vi "Logger.PGSQL.TestLauncher.vi"() -> ()   [LabVIEW 2019, in "Logger.PGSQL.lvclass"]
uses:
  Logger.PGSQL.lvclass
  <vilib>/JKI/JKI SMO/SMO/Typedefs/SMOState --Enum.ctl
  C:/Program Files (x86)/National Instruments/LabVIEW 2019/vi.lib/JKI/JKI SMO/SMO/SMO.lvclass
  C:/Users/patrick/Documents/GitHub/Instrument-Framework/lvsrc/SMOs/Logger/Logger.lvclass
  <vilib>/JKI/JKI SMO/SMO/SMO.lvclass/SMO.ctl
  <vilib>/JKI/JKI SMO/SMO/Private/ReftoDVR--SMO.vi
  <vilib>/JKI/JKI SMO/SMO/SMO.lvclass
  Logger/Logger.lvclass
panel:
  out "Data":variant
  out "x+1":i32=3
  out "time":u32
  out "read":u32
  out "write":u32=341910847
  in  "Address":string="llab_038:d005(TEST_TABLE--Columntest2())"
  in  "Write":bool
  in  "test value":dbl=2.0
  out "SMO State":T1=enum."Stopped"
  out "error out":errorcluster
  in  "Stop":bool
  # "Logger Test Launcher (postgreSQL)"
  # "For instructions on how to use the JKI State Machine Objects, examples and video tutorials, visit:\nhttp://jki.net/state-machine-objects/\n\nJKI State Machine Objects™\nhttp://jki.net/state-machine-objects/\nCopyright (C) 2005-2015, JKI <info@jki.net>\nALL RIGHTS RESERVED"
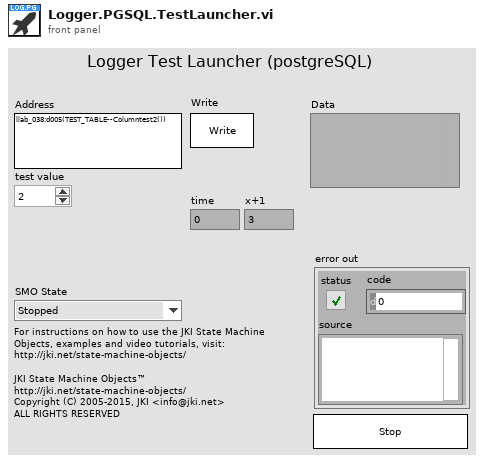
[diagram p1: front panel]
types:
  T1 = typedef "SMO.lvclass/SMOState --Enum.ctl" = enum16{"unknown", "Created", "Started", "Stopped"}
  T2 = typedef "SMO.lvclass/Public Events.ctl" = cluster{"Error":refnum<user-event>, "State":refnum<user-event>, "Reserve State":refnum<user-event>}
  T3 = typedef "Logger.PGSQL.lvclass/PublicEvents--Cluster.ctl" = cluster{"Read Variable":refnum<user-event>}
  T4 = cluster{"Event Registration Refnum":refnum<event-registration>}
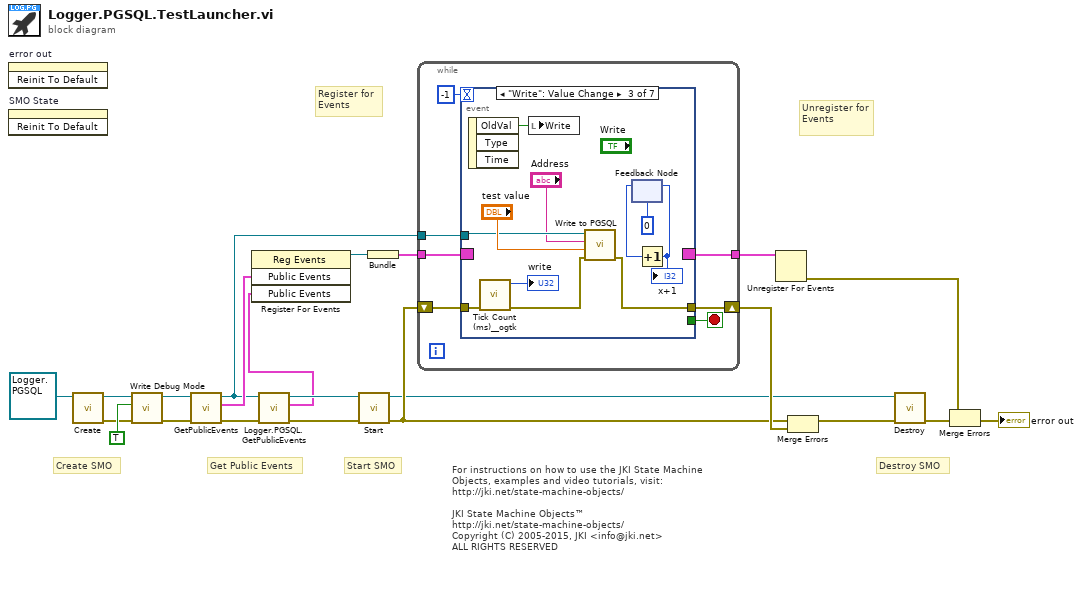
[diagram p0: block diagram]
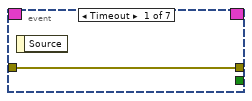
[diagram p2: hidden frame]
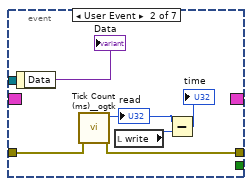
[diagram p3: hidden frame]
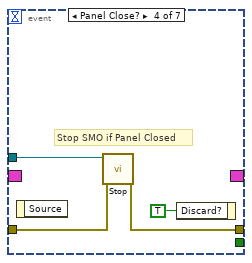
[diagram p4: hidden frame]
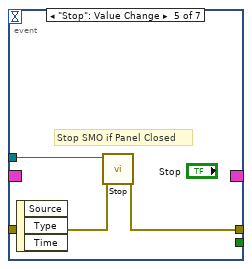
[diagram p5: hidden frame]
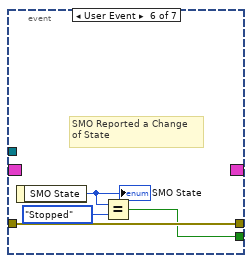
[diagram p6: hidden frame]
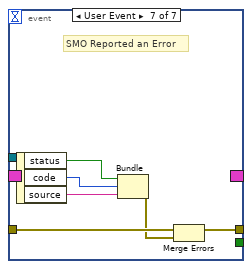
[diagram p7: hidden frame]
diagram:
  # "For instructions on how to use the JKI State Machine Objects, examples and video tutorials, visit:\nhttp://jki.net/state-machine-objects/\n\nJKI State Machine Objects™\nhttp://jki.net/state-machine-objects/\nCopyright (C) 2005-2015, JKI <info@jki.net>\nALL RIGHTS RESERVED"
  # "Get Public Events"
  # "Start SMO"
  # "Destroy SMO"
  # "Create SMO"
  # "Unregister for Events"
  # "Register for Events"
  n1 = invoke on="error out" class="Clust (strict)" method="Reinit To Default"() -> ()  [unwired: 3 in, 3 out]
  n2 = invoke on="SMO State" class="Enum (strict)" method="Reinit To Default"() -> ()  [unwired: 3 in, 3 out]
  n3 = call <vilib>:"Create.vi"("SMO"=refnum<class "Logger.PGSQL.lvclass"> refnum ("SMO.Template.lvclass")) -> ("error out"=w4:errorcluster, "SMO out"=w1:refnum<class "Logger.PGSQL.lvclass">)  [unwired: 8 in, 1 out]
  n4 = call "Write Debug Mode.vi"("error in (no error)"=w4, "Debug Mode?"=TRUE, "Logger in"=w1) -> ("error out"=w3:errorcluster, "Logger out"=w2:refnum<class "Logger.PGSQL.lvclass">)  [unwired: 7 in]
  n5 = call <vilib>:"GetPublicEvents.vi"("error in (no error)"=w3, "SMO"=w2) -> ("error out"=w9:errorcluster, "Public Events"=w12:T2, "SMO out"=w10:refnum<class "Logger.PGSQL.lvclass">)  [unwired: 7 in]
  n6 = call "Logger.PGSQL.GetPublicEvents.vi"("error in (no error)"=w9, "Logger"=w10) -> ("error out"=w8:errorcluster, "Public Events"=w6:T3, "Logger out"=w7:refnum<class "Logger.PGSQL.lvclass">)  [unwired: 7 in]
  n7 = register-events(w12, w6) -> (reference out=w11:refnum<event-registration>)  [unwired: 2 in, 1 out]
  n8 = call <vilib>:"Start.vi"("error in (no error)"=w8, "SMO"=w7) -> ("error out"=w15:errorcluster, "SMO out"=w13:refnum<class "Logger.PGSQL.lvclass">)  [unwired: 8 in]
  n9 = Bundle("Event Registration Refnum"=w11) -> (w21:T4)  [unwired: 1 in]
  n10 = while {
    shift-right: [w28] -> w20
    shift-left: w15 -> [w27]
    tunnel: w21 -> [w26]
    tunnel: [w25] -> w22
    tunnel: w10 -> [w24]
    stop <- w29 stop-if-true
    n11 = event shown="[2] \"Write\": Value Change" {
      selector: w26 -> [_ _ _ _ _ _ _]
      dyn-events: [_ _ _ _ _ _ _] -> w25
      timeout: -1 -> [_ _ _ _ _ _ _]
      tunnel: [_ _ _ _ _ w55 _] -> w29
      tunnel: w24 -> [_ _ w38 w51 w54 _ _]
      tunnel: [w30 w35 w39 w50 w53 w58 w62] -> w28
      tunnel: w27 -> [w30 w36 w47 w49 w52 w58 w60]
      event Timeout {
        n12 = event-data() -> ()  [unwired: 1 in, 1 out]
      }
      event User Event {
        n13 = event-data() -> ("Data"=→"Data":variant)  [unwired: 1 in]
        n14 = call <userlib>:"Tick Count (ms)__ogtk.vi"("error in (no error)"=w36) -> ("error out"=w35:errorcluster, "millisecond timer value"=w33:u32)  [unwired: 9 in]
        "read" <- w33
        n15 = local read "write"() -> (w34:u32)
        n16 = Subtract(x=w33, y=w34) -> (x-y=→"time":u32)
      }
      event "Write": Value Change {
        n17 = event-data() -> ("OldVal"=w42:bool)  [unwired: 1 in, 2 out]
        n18 = call <userlib>:"Tick Count (ms)__ogtk.vi"("error in (no error)"=w47) -> ("error out"=w40:errorcluster, "millisecond timer value"=→"write":u32)  [unwired: 9 in]
        n19 = local write "Write"(w42) -> ()
        n20 = call-dynamic "Write to PGSQL.vi"("error in (no error)"=w40, "Variant"="test value", "Path"="Address", "Logger in"=w38) -> ("error out"=w39:errorcluster)  [unwired: 6 in, 1 out]
        n21 = feedback #1(0) -> (w44:i32)
        n22 = Increment(x=w44) -> (x+1=w45:i32)
        "x+1" <- w45
        n23 = feedback-in #1(w45) -> ()
      }
      event Panel Close? {
        # "Stop SMO if Panel Closed"
        n24 = event-data() -> ()  [unwired: 1 in, 1 out]
        n25 = call <vilib>:"Stop.vi"("error in (no error)"=w49, "SMO"=w51) -> ("error out"=w50:errorcluster)  [unwired: 8 in, 1 out]
        n26 = event-data("Discard?"=TRUE ("OK")) -> ()  [unwired: 1 in, 1 out]
      }
      event "Stop": Value Change {
        # "Stop SMO if Panel Closed"
        n27 = event-data() -> ()  [unwired: 1 in, 3 out]
        n28 = call <vilib>:"Stop.vi"("error in (no error)"=w52, "SMO"=w54) -> ("error out"=w53:errorcluster)  [unwired: 8 in, 1 out]
      }
      event User Event {
        # "SMO Reported a Change\nof State"
        n29 = event-data() -> ("SMO State"=w57:T1)  [unwired: 1 in]
        "SMO State" <- w57
        n30 = Equal?(x=w57, y=SMOState_--Enum."Stopped") -> (x = y?=w55:bool)
      }
      event User Event {
        # "SMO Reported an Error"
        n31 = event-data() -> ("status"=w61:bool, "code"=w64:i32, "source"=w63:string)  [unwired: 1 in]
        n32 = Bundle("status"=w61, "code"=w64, "source"=w63) -> (w59:errorcluster)  [unwired: 1 in]
        n33 = Merge Errors(w60, w59) -> (w62:errorcluster)
      }
    }
  }
  n34 = Unregister For Events(event registration refnum=w22) -> (error out=w19:errorcluster)  [unwired: 1 in]
  n35 = Merge Errors(w15, w20) -> (w14:errorcluster)
  n36 = call <vilib>:"Destroy.vi"("error in (no error)"=w14, "SMO"=w13) -> ("error out"=w17:errorcluster)  [unwired: 9 in]
  n37 = Merge Errors(w19, w17) -> (→"error out":errorcluster)
